vi "2-Odd Integer Search.vi"() -> ()   [LabVIEW 2014]
panel:
  out "Smallest Odd Integer":dbl
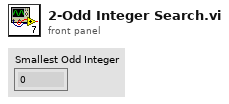
[diagram p1: front panel]
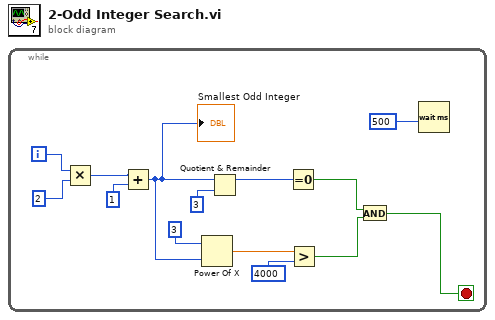
[diagram p0: block diagram]
diagram:
  n1 = while {
    i -> [w14]
    stop <- w10 stop-if-true
    n2 = Multiply(x=w14, y=2) -> (x*y=w11:i32)
    n3 = Add(x=w11, y=1) -> (x+y=w3:i32)
    "Smallest Odd Integer" <- w3
    n4 = Power Of X(1:w3, 2:3) -> (0:w8:dbl)
    n5 = Quotient & Remainder(x=w3, y=3) -> (x-y*floor(x/y)=w2:i32)  [unwired: 1 out]
    n6 = Equal To 0?(x=w2) -> (x = 0?=w1:bool)
    n7 = Greater?(x=w8, y=4000) -> (0:w6:bool)
    n8 = And(x=w1, y=w6) -> (x .and. y?=w10:bool)
    n9 = Wait (ms)(milliseconds to wait=u32 500 ("millisecond timer value")) -> ()  [unwired: 1 out]
  }
